vi "02passwordcoder-SIMPLE.vi"(3 "retein":bool caption="Recordar contraseña", 4 "pass":string="0891", 5 "name":string="admin") -> (0 "OK":bool, 1 "retein 2":bool caption="Recordar contraseña")   [LabVIEW 2010]
panel:
  in  "change":bool
  out "error!":bool=TRUE
  in  "CANC":bool
  in  "Nombre:":string
  in  "aceptar":bool
  in  "Contraseña:":string
  # "INGRESE:\nNOMBRE Y CONTRASEÑA"
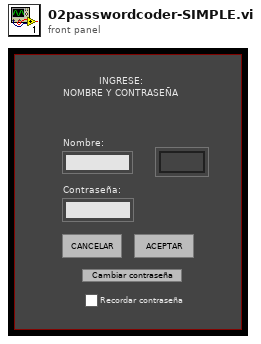
[diagram p1: front panel]
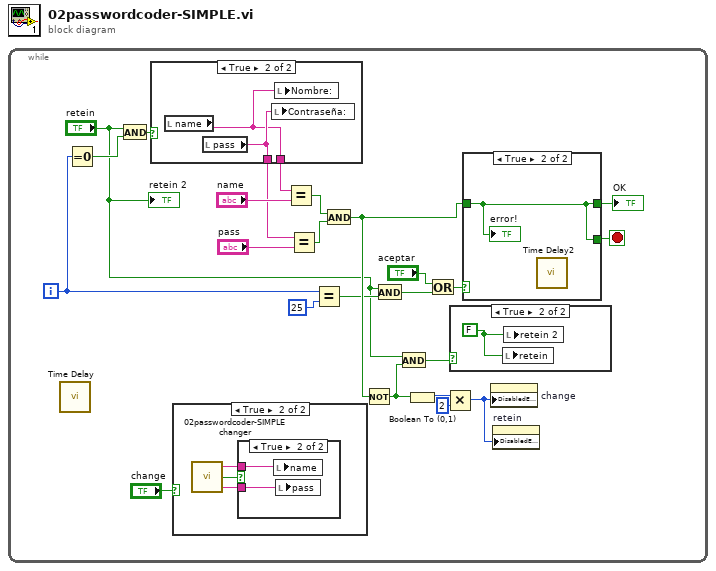
[diagram p0: block diagram]
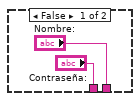
[diagram p3: hidden frame]
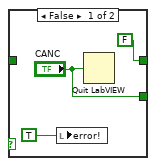
[diagram p6: hidden frame]
diagram:
  n1 = while {
    i -> [w6]
    stop <- w24 stop-if-true
    n2 = call "Time Delay"() -> ()  [unwired: 11 in, 1 out]
    n3 = Equal To 0?(x=w6) -> (x = 0?=w5:bool)
    n4 = And(x="retein", y=w5) -> (x .and. y?=w4:bool)
    n5 = case shown="True" w4 {
      tunnel: ["Contraseña:" w29] -> w12
      tunnel: ["Nombre:" w28] -> w11
      frame False {
      }
      frame True {
        n6 = local read "name"() -> (w28:string)
        n7 = local read "pass"() -> (w29:string)
        n8 = local write "Contraseña:"(w29) -> ()
        n9 = local write "Nombre:"(w28) -> ()
      }
    }
    n10 = case shown="True" "change" {
      frame False {
      }
      frame True {
        n11 = call "02passwordcoder-SIMPLEchanger.vi"() -> ("pass"=w31:string, "Boolean"=w30:bool, "name"=w32:string)  [unwired: 3 in]
        n12 = case shown="True" w30 {
          tunnel: w32 -> [_ w34]
          tunnel: w31 -> [_ w33]
          frame False {
          }
          frame True {
            n13 = local write "name"(w34) -> ()
            n14 = local write "pass"(w33) -> ()
          }
        }
      }
    }
    n15 = Equal?(x=w11, y="name") -> (x = y?=w19:bool)
    n16 = Equal?(x=w12, y="pass") -> (x = y?=w18:bool)
    n17 = Equal?(x=w6, y=25) -> (x = y?=w8:bool)
    n18 = And(x=w19, y=w18) -> (x .and. y?=w13:bool)
    n19 = Not(x=w13) -> (.not. x?=w3:bool)
    n20 = And(x="retein", y=w8) -> (x .and. y?=w7:bool)
    n21 = And(x="retein", y=w3) -> (x .and. y?=w1:bool)
    n22 = Boolean To (0,1)(Boolean=w3) -> (0, 1=w15:i16)
    n23 = Or(x="aceptar", y=w7) -> (x .or. y?=w23:bool)
    n24 = Multiply(x=w15, y=i16 2) -> (x*y=w10:i16)
    n25 = case shown="True" w1 {
      frame False {
      }
      frame True {
        w25 = FALSE ("retein")
        n26 = local write "retein"(w25) -> ()
        n27 = local write "retein 2"(w25) -> ()
      }
    }
    n28 = case shown="True" w23 {
      tunnel: w13 -> [_ w38]
      tunnel: ["CANC" w38] -> w24
      tunnel: [FALSE w38] -> w17
      frame False {
        n29 = local write "error!"(TRUE) -> ()
        n30 = Quit LabVIEW(quit? (T)="CANC") -> ()
      }
      frame True {
        n31 = call "Time Delay2"() -> ()  [unwired: 11 in, 1 out]
        "error!" <- w38
      }
    }
    "OK" <- w17
    n32 = property on="change" class="Bool"("DisabledEnum"=w10) -> ()  [unwired: 2 in, 2 out]
    n33 = property on="retein" class="Bool (strict)"("DisabledEnum"=w10) -> ()  [unwired: 2 in, 2 out]
    "retein 2" <- "retein"
  }
